vi "Field.vi"(4 "channel 2":T3, 6 "Draw Targets?":T2, 7 "AutoScale":bool=TRUE, 8 "IA State Output":T4, 10 "Scale mm/pixel":dbl=1.0 format="%#_13g", 11 "channel":T1) -> (2 "Scale Out":dbl, 3 "2D Picture":picture, 5 "AutoScale Out":bool=TRUE)   [LabVIEW 2017]
uses:
  <extravilib>/ChannelInstances/Lossy Stream-a[.](i32)/)Channel.ctl
  DrawTargets.ctl
  <extravilib>/ChannelInstances/Lossy Stream-t'SSL Field State.ctl'/)Channel.ctl
  SSL/SSL Field State.ctl
  SSL Detection Frame.ctl
  SSL Detection Robot.ctl
  <vilib>/Analysis/Matrix/Datatypes/RealMatrix.ctl
  SSL Detection Ball.ctl
  Core/AI Input.ctl
  Core/AI Robot.ctl
  Intel/Functions Enum.ctl
  Intel/AttackerStates.ctl
  Path Planning/RRT/PathDests.ctl
  Path Planning/RRT/PathDest.ctl
  Core/AI Ball.ctl
  Core/Field Size.ctl
  Core/AI Judge.ctl
  Intel/Command Enum.ctl
  Util/Events/Events.ctl
  <vilib>/Utility/miscctls.llb/LVBoundsTypeDef.ctl
  <extravilib>/ChannelInstances/Lossy Stream-t'SSL Field State.ctl'/Read With Abort.vi
  <extravilib>/ChannelInstances/Lossy Stream-a[.](i32)/Read With Abort.vi
  <extravilib>/ChannelInstances/Lossy Stream-t'SSL Field State.ctl'/EndpointRead.vi
  <extravilib>/ChannelInstances/Lossy Stream-a[.](i32)/EndpointRead.vi
  <extravilib>/ChannelInstances/Lossy Stream-a[.](i32)/)Channel.vi
  <resource>/ChannelSupport/_ChannelSupport/WaitIfNeeded.vi
  <extravilib>/ChannelInstances/Lossy Stream-t'SSL Field State.ctl'/)Channel.vi
  <extravilib>/ChannelInstances/Lossy Stream-a[.](i32).lvlib
  <extravilib>/ChannelInstances/Lossy Stream-t'SSL Field State.ctl'.lvlib
  <vilib>/Analysis/Matrix/NI_Matrix.lvlib
panel:
  in  "Draw Number":bool=TRUE
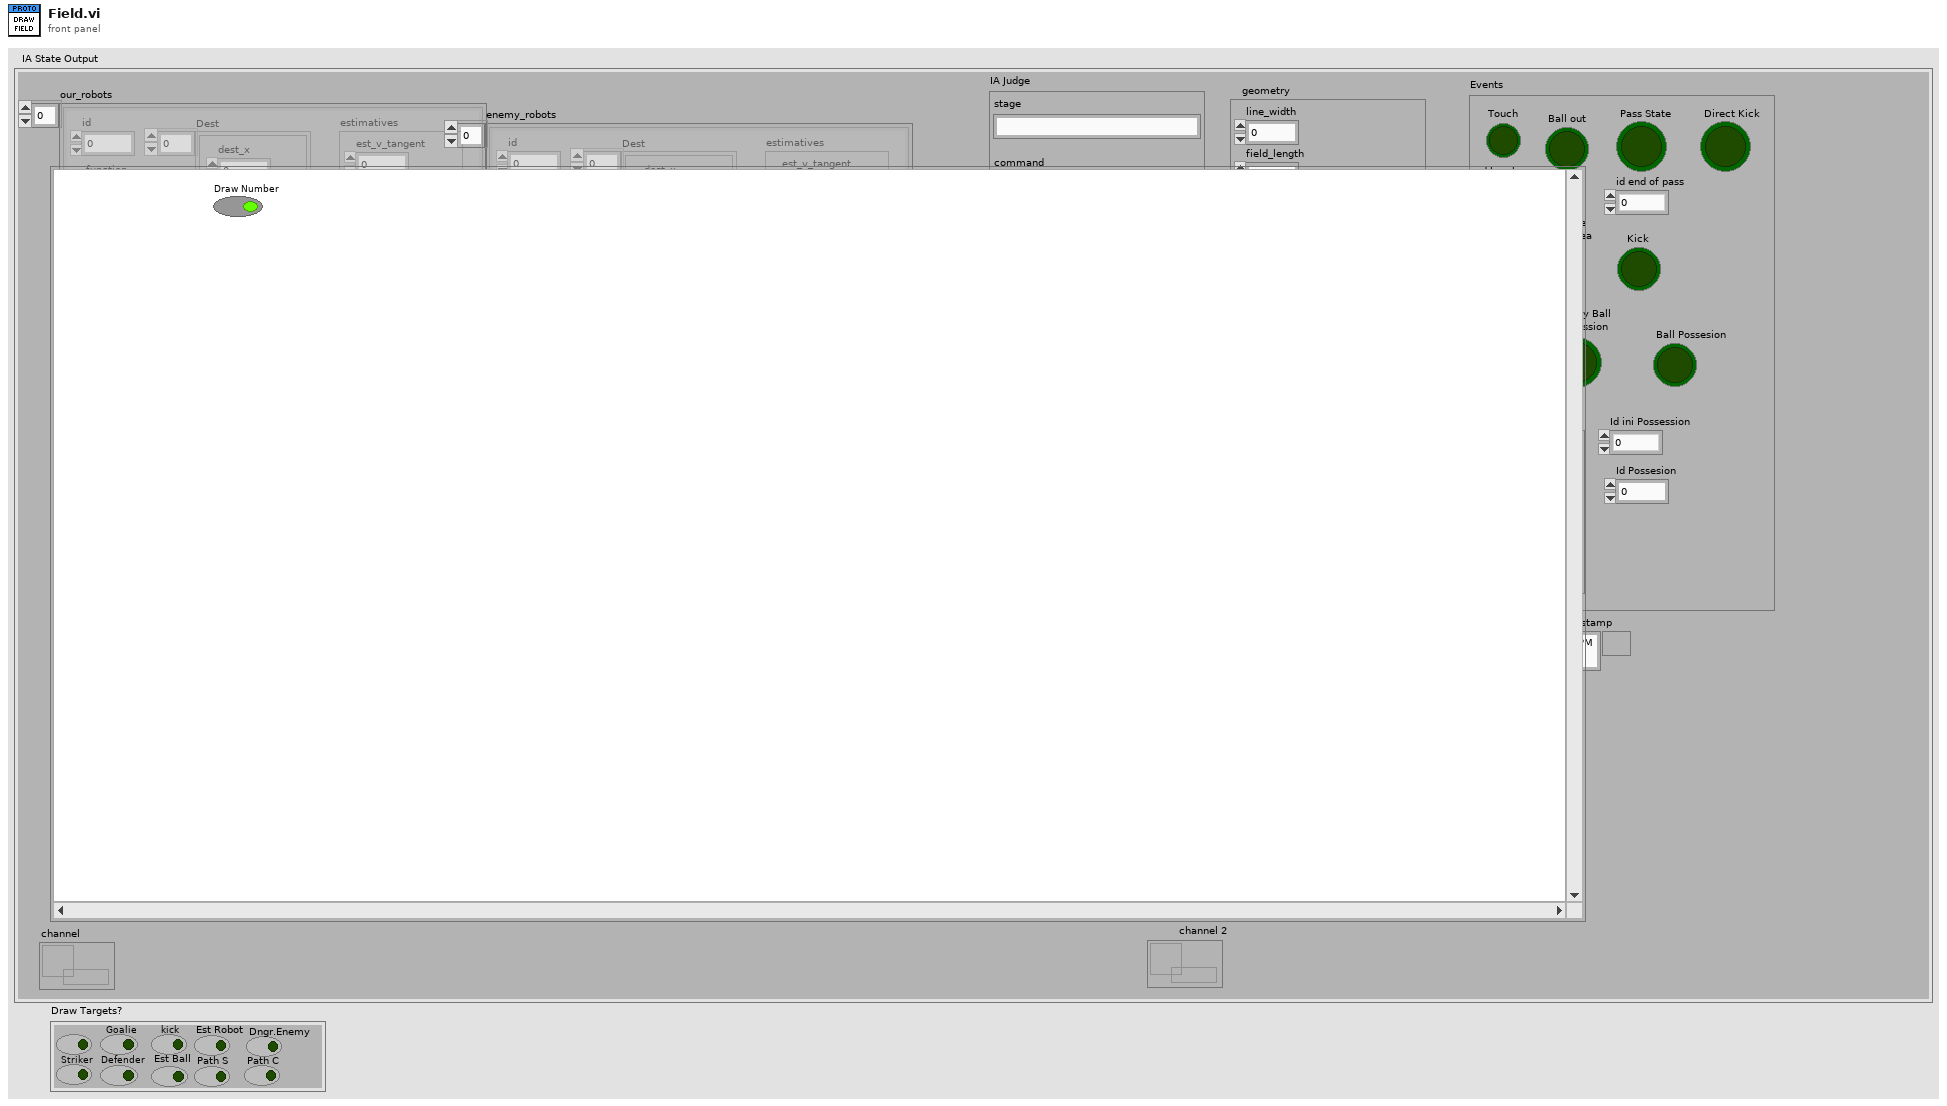
[diagram p1: front panel]
types:
  T1 = typedef "Lossy Stream-t'SSL Field State.ctl'.lvlib/)Channel.ctl" = refnum<queue>
  T2 = typedef "DrawTargets.ctl" = cluster{"Attacker":bool, "Striker":bool, "Goalie":bool, "Defender":bool, "kick":bool, "Est Ball":bool, "Est Robot":bool, "Path S":bool, "Path C":bool, "Dngr.Enemy":bool}
  T3 = typedef "Lossy Stream-a[.](i32).lvlib/)Channel.ctl" = refnum<queue>
  T4 = typedef "AI Input.ctl" = cluster{"our_robots":T5[], "enemy_robots":T5[], "balls":T10[], "geometry":T11, "IA Judge":T12, "Received Timestamp":timestamp, "Events":T14}
  T5 = typedef "AI Robot.ctl" = cluster{"id":u32, "function":T6, "x":dbl, "y":dbl, "orientation":dbl, "v_tangent":dbl, "v_normal":dbl, "v_ang":dbl, "kick_x":dbl, "kick_z":dbl, "dribble":bool, "Timestamp":timestamp, "estimatives":cluster{"est_v_tangent":dbl, "est_v_normal":dbl, "est_vx":dbl, "est_vy":dbl, "Pos Robot Est":dbl[]}, "dest_x_kick":dbl, "dest_y_kick":dbl, "Gap Coord":dbl[], "States":T7, "Path ":dbl[][], "Path  Smooth":dbl[][], "Dest":T8}
  T6 = typedef "Functions Enum.ctl" = enum16{"Attacker", "Goalie", "Defender", "Striker", "Goto 0", "Dummy", "Kicker", "ZigZag 0", "ZigZag 1", "ZigZag 2", "ZigZag 3", "ZigZag 4", "ZigZag 5", "ZigZag 6", "ZigZag 7", "ZigZag 8", ""}
  T7 = typedef "AttackerStates.ctl" = enum16{"Pass", "GoToTangent", "BallGetting", "GoToKick", ""}
  T8 = typedef "PathDests.ctl" = T9[]
  T9 = typedef "PathDest.ctl" = cluster{"dest_x":dbl, "dest_y":dbl, "dest_orientation":dbl, "dest_vel":dbl}
  T10 = typedef "AI Ball.ctl" = cluster{"x":dbl, "y":dbl, "timestamp":timestamp, "Vel_x":dbl, "Vel_y":dbl, "Pos Bola Est":dbl[]}
  T11 = typedef "Field Size.ctl" = cluster{"line_width":u32, "field_length":u32, "field_width":u32, "boundary_width":u32, "referee_width":u32, "goal_width":u32, "goal_depth":u32, "goal_wall_width":u32, "center_circle_radius":u32, "defense_radius":u32, "defense_stretch":u32, "free_kick_from_defense_dist":u32, "penalty_spot_from_field_line_dist":u32, "penalty_line_from_spot_dist":u32}
  T12 = typedef "AI Judge.ctl" = cluster{"stage":string, "command":string, "our_goalie_id":dbl, "enemy_goalie_id":dbl, "command enum":T13, "Time":enum16{"Azul", "Amarelo"}}
  T13 = typedef "Command Enum.ctl" = enum16{"Halt", "Stop", "Force Start", "PKA Normal Start", "Prepare Kickoff Ally", "PKE Normal Start", "Prepare Kickoff Enemy", "Prepare Penalty Ally", "PPA Normal Start", "Prepare Penalty Enemy", "PPE Normal Start", "Direct Free Enemy", "Direct Free Ally", "Indirect Free Enemy", "Indirect Free Ally", "Timeout Enemy", "Timeout Ally", "Goal Enemy", "Goal Ally", "Ball Placement Enemy", "Ball Placement Ally", "Normal Half Time", "Extra Time Break", "Extra Half Time", "None", "Post Game"}
  T14 = typedef "Events.ctl" = cluster{"Touch":bool, "Ball out":bool, "id touch":dbl, "Ball out of \nVision":bool, "Ball inside \nGoalie area":bool, "Robot not responding":bool, "Robots responding status":dbl[], "Enemy Ball \nPossession":bool, "Pass State":bool, "id end of pass":dbl, "Kick":bool, "Id ini Possession":dbl, "Ball Possesion":bool, "Id Possesion":dbl, "Direct Kick":bool}
  T15 = typedef "LVBoundsTypeDef.ctl" = cluster{"Width":u32, "Height":u32}
  T16 = typedef "SSL Field State.ctl" = cluster{"Detection Frame Out":T17, "Field Size Out":cluster{"line_width":u32, "field_length":u32, "field_width":u32, "boundary_width":u32, "referee_width":u32, "goal_width":u32, "goal_depth":u32, "goal_wall_width":u32, "center_circle_radius":u32, "defense_radius":u32, "defense_stretch":u32, "free_kick_from_defense_dist":u32, "penalty_spot_from_field_line_dist":u32, "penalty_line_from_spot_dist":u32}, "Received Time Stamp":timestamp}
  T17 = typedef "SSL Detection Frame.ctl" = cluster{"frame_number":u32, "t_capture":dbl, "t_sent":dbl, "camera_id":u32, "robots_yellow":T18[], "robots_blue":T18[], "balls":T20[], "Valid":bool, "Time Stamp":timestamp}
  T18 = typedef "SSL Detection Robot.ctl" = cluster{"x":sgl, "robot_id":u32, "confidence":sgl, "y":sgl, "orientation":sgl, "pixel_x":sgl, "pixel_y":sgl, "height":sgl, "Valid":bool, "Time Stamp":timestamp, "x_k|k":T19, "Pk|k":T19, "Previous Time Stamp":timestamp, "R":T19}
  T19 = typedef "NI_Matrix.lvlib/RealMatrix.ctl" = dbl[][]
  T20 = typedef "SSL Detection Ball.ctl" = cluster{"x":sgl, "area":u32, "confidence":sgl, "y":sgl, "z":sgl, "pixel_x":sgl, "pixel_y":sgl, "Valid":bool, "Time Stamp":timestamp, "x_k|k":T19, "Pk|k":T19, "Id":u32, "Previous Time Stamp":timestamp, "R":T19}
  T21 = cluster{"line_width":u32, "field_length":u32, "field_width":u32, "boundary_width":u32, "referee_width":u32, "goal_width":u32, "goal_depth":u32, "goal_wall_width":u32, "center_circle_radius":u32, "defense_radius":u32, "defense_stretch":u32, "free_kick_from_defense_dist":u32, "penalty_spot_from_field_line_dist":u32, "penalty_line_from_spot_dist":u32}
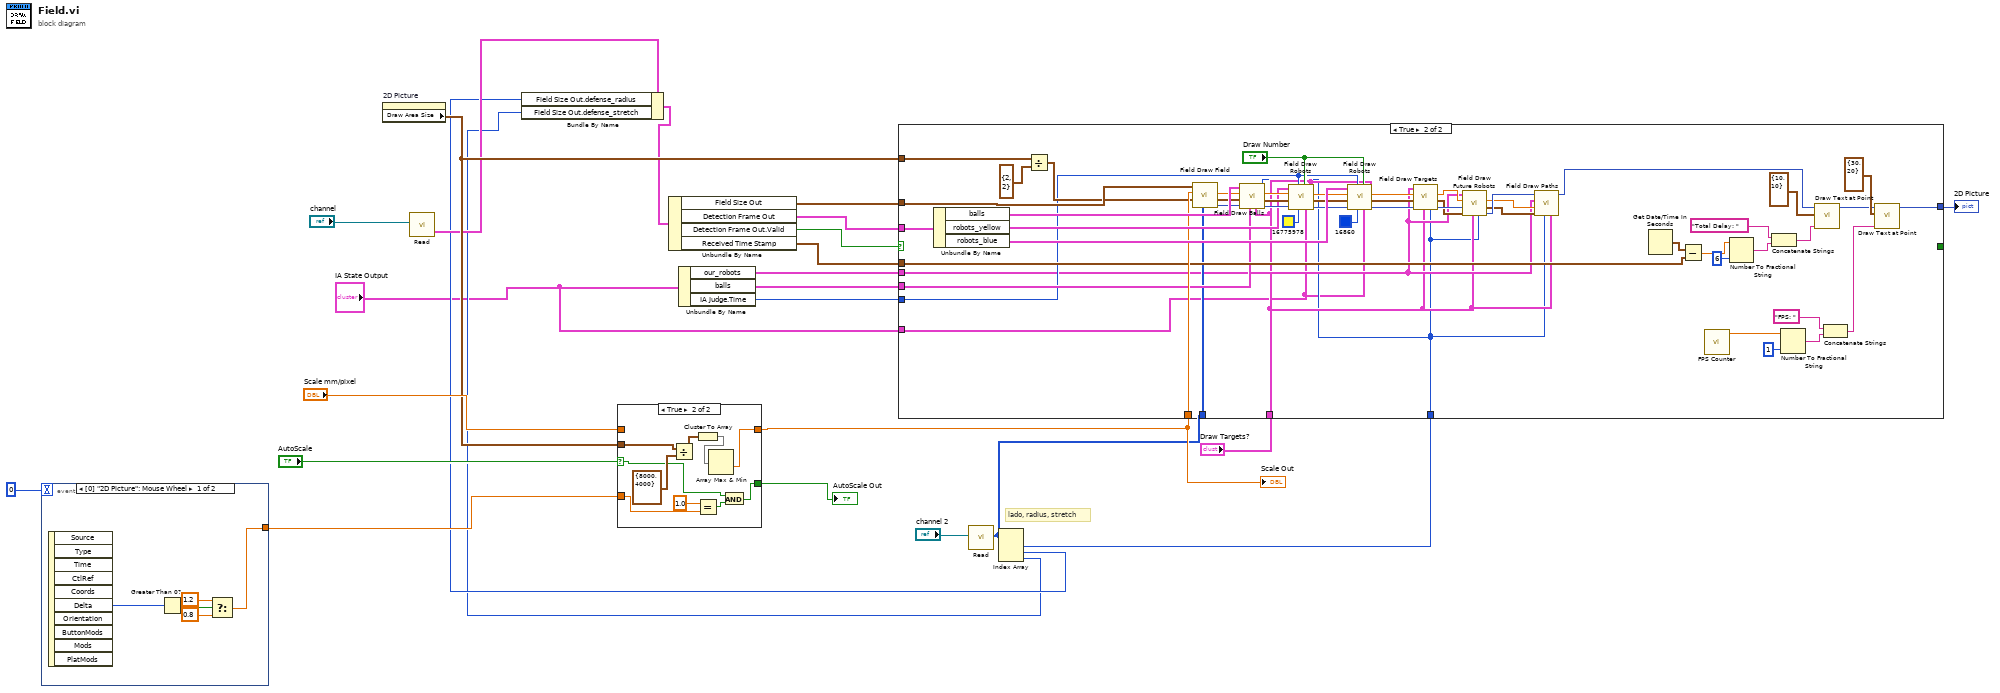
[diagram p0: block diagram]
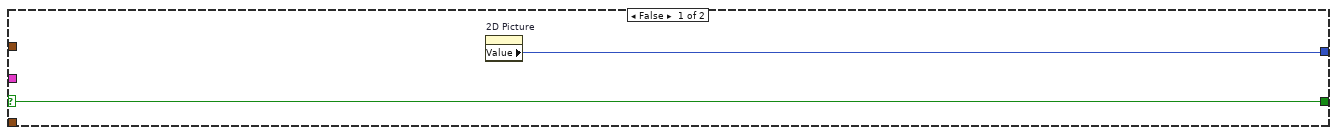
[diagram p2: hidden frame]
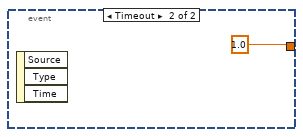
[diagram p3: hidden frame]
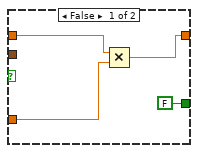
[diagram p4: hidden frame]
diagram:
  # "lado, radius, stretch"
  n1 = event shown="[0] \"2D Picture\": Mouse Wheel" {
    selector: _ -> [_ _]
    dyn-events: _ -> [_ _]
    timeout: 0 -> [_ _]
    tunnel: [w26 1.0] -> w23
    event "2D Picture": Mouse Wheel {
      n2 = event-data() -> ("Delta"=w30:i32)  [unwired: 1 in, 9 out]
      n3 = Greater Than 0?(x=w30) -> (x > 0?=w29:bool)
      n4 = Select(t=1.2, s=w29, f=0.8) -> (s? t:f=w26:dbl)
    }
    event Timeout {
      n5 = event-data() -> ()  [unwired: 1 in, 3 out]
    }
  }
  n6 = property on="2D Picture" class="Pict"() -> ("Draw Area Size"=w22:T15)  [unwired: 2 in, 2 out]
  n7 = call <extravilib>:"Read.vi"("channel"="channel") -> ("element"=w5:T16)  [unwired: 5 in, 5 out]
  n8 = case shown="True" "AutoScale" {
    selector: "AutoScale" -> [_ w37]
    tunnel: "Scale mm/pixel" -> [w35 _]
    tunnel: [w34 w41] -> w17
    tunnel: w22 -> [_ w45]
    tunnel: w23 -> [w33 w40]
    tunnel: [FALSE w38] -> w20
    frame False {
      n9 = Multiply(x=w35, y=w33) -> (x*y=w34:dbl)
    }
    frame True {
      n10 = Divide(x=w45, y=T15 {"Width"=8000, "Height"=4000}) -> (x/y=w43:cluster{"Width":dbl, "Height":dbl})
      n11 = Cluster To Array(cluster=w43) -> (array=w42:dbl[])
      n12 = Equal?(x=1.0, y=w40) -> (x = y?=w36:bool)
      n13 = Array Max & Min(array=w42) -> (min value=w41:dbl)  [unwired: 3 out]
      n14 = And(x=w37, y=w36) -> (x .and. y?=w38:bool)
    }
  }
  "Scale Out" <- w17
  "AutoScale Out" <- w20
  n15 = Unbundle By Name("IA State Output") -> ("our_robots"=w7:T5[], "balls"=w11:T10[], "IA Judge.Time"=w8:enum16{"Azul", "Amarelo"})
  n16 = call <extravilib>:"Read.vi"("channel"="channel 2") -> ("element"=w9:i32[])  [unwired: 5 in, 5 out]
  n17 = Index Array(array=w9) -> (element #1=w14:i32, element #2=w4:i32, element #3=w3:i32)  [unwired: 3 in]
  n18 = Bundle By Name(cluster=w5, "Field Size Out.defense_radius"=w4, "Field Size Out.defense_stretch"=w3) -> (w2:T16)
  n19 = Unbundle By Name(w2) -> ("Field Size Out"=w18:T21, "Detection Frame Out"=w19:T17, "Detection Frame Out.Valid"=w16:bool, "Received Time Stamp"=w15:timestamp)
  n20 = case shown="True" w16 {
    selector: w16 -> [w47 _]
    tunnel: w22 -> [_ w100]
    tunnel: [w46 w73] -> w13
    tunnel: w19 -> [_ w88]
    tunnel: w18 -> [_ w87]
    tunnel: w17 -> [_ w86]
    tunnel: [w47 _] -> _
    tunnel: w15 -> [_ w80]
    tunnel: w7 -> [_ w52]
    tunnel: "Draw Targets?" -> [_ w51]
    tunnel: w14 -> [_ w49]
    tunnel: w11 -> [_ w63]
    tunnel: w9 -> [_ w57]
    tunnel: w8 -> [_ w56]
    tunnel: "IA State Output" -> [_ w48]
    frame False {
      n21 = property on="2D Picture" class="Pict"() -> ("Value"=w46:picture)  [unwired: 2 in, 2 out]
    }
    frame True {
      n22 = Unbundle By Name(w88) -> ("balls"=w99:T20[], "robots_yellow"=w95:T18[], "robots_blue"=w94:T18[])
      n23 = Divide(x=w100, y=T15 {"Width"=2, "Height"=2}) -> (x/y=w83:cluster{"Width":dbl, "Height":dbl})
      n24 = call "Field Draw Field.vi"("Lado,radius, stretch"=w57, "Offset"=w83, "Scale"=w86, "Field Size"=w87) -> ("new picture out"=w84:picture, "Offset Out"=w82:cluster{"Width":dbl, "Height":dbl}, "Scale Out"=w85:dbl)  [unwired: 5 in]
      n25 = call "Field Draw Balls.vi"("Lado"=w49, "Draw Targets?"=w51, "balls"=w63, "Picture In"=w84, "Offset"=w82, "Scale"=w85, "Balls"=w99) -> ("Picture Out"=w98:picture, "Offset Out"=w97:cluster{"Width":dbl, "Height":dbl}, "Scale Out"=w96:dbl)  [unwired: 2 in]
      n26 = call "Field Draw Robots.vi"("Draw Targets?"=w51, "IA state"=w48, "Draw Number"="Draw Number", "color(black)"=u32 16775978, "IA Judge.Time"=w56, "Picture In"=w98, "Offset"=w97, "Scale"=w96, "Detection Robots"=w95) -> ("Picture Out"=w91:picture, "Offset Out"=w92:cluster{"Width":dbl, "Height":dbl}, "Scale Out"=w93:dbl)
      n27 = call "Field Draw Robots.vi"("Draw Targets?"=w51, "IA state"=w48, "Draw Number"="Draw Number", "color(black)"=u32 16860, "IA Judge.Time"=w56, "Picture In"=w91, "Offset"=w92, "Scale"=w93, "Detection Robots"=w94) -> ("Picture Out"=w65:picture, "Offset Out"=w64:cluster{"Width":dbl, "Height":dbl}, "Scale Out"=w62:dbl)
      n28 = call "Field Draw Targets.vi"("Lado"=w49, "Draw Targets?"=w51, "Picture In"=w65, "Offset"=w64, "Scale"=w62, "our_robots"=w52) -> ("Picture Out"=w61:picture, "Offset Out"=w60:cluster{"Width":dbl, "Height":dbl}, "Scale Out"=w59:dbl)  [unwired: 3 in]
      n29 = call "Field Draw Future Robots.vi"("Lado"=w49, "Draw Targets?"=w51, "Offset"=w60, "Picture In"=w61, "Scale"=w59, "our_robots"=w52) -> ("Picture Out"=w55:picture, "Offset Out"=w53:cluster{"Width":dbl, "Height":dbl}, "Scale Out"=w54:dbl)  [unwired: 3 in]
      n30 = call "Field Draw Paths.vi"("Draw Targets?"=w51, "Lado"=w49, "Offset"=w53, "Scale mm/pixel"=w54, "our_robots"=w52, "picture in"=w55) -> ("picture out"=w50:picture)  [unwired: 5 in]
      n31 = Get Date/Time In Seconds() -> (seconds since 1Jan1904=w79:timestamp)
      n32 = Subtract(x=w79, y=w80) -> (x-y=w78:dbl)
      n33 = call "FPS Counter.vi"() -> ("Numeric"=w69:dbl)  [unwired: 11 in]
      n34 = Number To Fractional String(number=w78, precision (6)=i16 6) -> (F-format string=w76:string)  [unwired: 2 in]
      n35 = Concatenate Strings("Total Delay: " ("text"), w76) -> (w75:string)
      n36 = Number To Fractional String(number=w69, precision (6)=i16 1) -> (F-format string=w71:string)  [unwired: 2 in]
      n37 = call <vilib>:"Draw Text at Point.vi"("text"=w75, "origin"=cluster{"x":i16, "y":i16} {"x"=10, "y"=10}, "picture"=w50) -> ("new picture"=w58:picture)  [unwired: 7 in, 1 out]
      n38 = Concatenate Strings("FPS: " ("text"), w71) -> (w67:string)
      n39 = call <vilib>:"Draw Text at Point.vi"("text"=w67, "origin"=cluster{"x":i16, "y":i16} {"x"=30, "y"=20}, "picture"=w58) -> ("new picture"=w73:picture)  [unwired: 7 in, 1 out]
    }
  }
  "2D Picture" <- w13
